vi "LNLS Control FOFB Configuration In.vi"() -> ()   [LabVIEW 2011, in "Controller Global Variables.lvlib"]
uses:
  Controller Global Variables.lvlib
panel:
  in  "LNLS Control FOFB Configuration In":T1
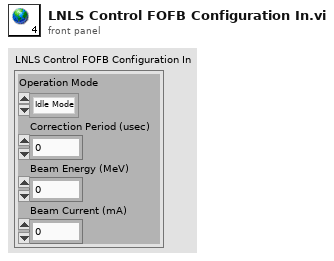
[diagram p1: front panel]
types:
  T1 = cluster{"Operation Mode":enum16{"Idle Mode", "Error Mode", "Manual Mode", "FOFB Mode", "RMM Mode"}, "Correction Period (usec)":i32, "Beam Energy (MeV)":sgl, "Beam Current (mA)":sgl}
diagram:
